vi "Read Work Space.vi"(3 "FP":refnum<class "FP.lvclass">) -> (1 "WkSpace Out":T1)   [LabVIEW 2020, in "FP.lvclass"]
uses:
  FP.lvclass
  <vilib>/Utility/miscctls.llb/LVRectTypeDef.ctl
  FP.lvclass/FP.ctl
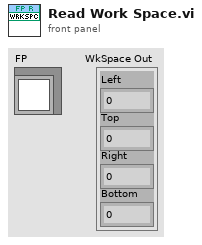
[diagram p1: front panel]
types:
  T1 = typedef "LVRectTypeDef.ctl" = cluster{"Left":i16, "Top":i16, "Right":i16, "Bottom":i16}
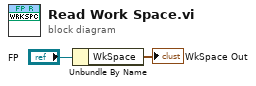
[diagram p0: block diagram]
diagram:
  n1 = Unbundle By Name("FP") -> ("WkSpace"=→"WkSpace Out":T1)
